vi "display_array.vi"(8 "array":i32[](array[numeric]), 11 "NXT":T1={"Hardware"="NXT", "Flattened String"=""}) -> (3 "NXT 2":T1={"Hardware"="NXT", "Flattened String"=""})   [LabVIEW 2012]
uses:
  <vilib>/NXT/Subs/LVHSConnector.ctl
  <vilib>/NXT/Dual Mode Library/Display/drawLine.vi
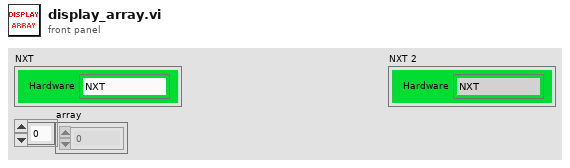
[diagram p1: front panel]
types:
  T1 = typedef "LVHSConnector.ctl" = cluster{"Hardware":string, "Flattened String":string}
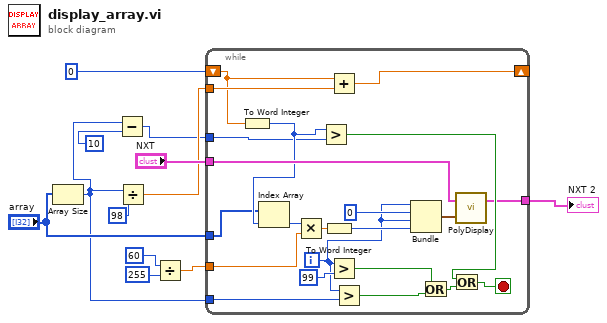
[diagram p0: block diagram]
diagram:
  n1 = Array Size(array="array") -> (size(s)=w2:i32)
  n2 = Subtract(x=w2, y=10) -> (x-y=w1:i32)
  n3 = Divide(x=w2, y=98) -> (x/y=w5:dbl)
  n4 = Divide(x=i16 60 ("Start X"), y=i16 255 ("Start X")) -> (x/y=w12:dbl)
  n5 = while {
    tunnel: [w13] -> w8
    tunnel: w12 -> [w32]
    tunnel: "NXT" -> [w29]
    tunnel: w5 -> [w28]
    shift-right: [w23] -> _
    shift-left: 0 -> [w24]
    tunnel: w2 -> [w14]
    tunnel: "array" -> [w17]
    tunnel: w1 -> [w15]
    i -> [w25]
    stop <- w19 stop-if-true
    n6 = To Word Integer(number=w24) -> (16bit integer=w22:i16)
    n7 = Index Array(array=w17, index=w22) -> (element=w16:i32)
    n8 = Multiply(x=w16, y=w32) -> (x*y=w34:dbl)
    n9 = Greater?(x=w22, y=w15) -> (0:w18:bool)
    n10 = To Word Integer(number=w34) -> (16bit integer=w31:i16)
    n11 = Add(x=w24, y=w28) -> (x+y=w23:dbl)
    n12 = Greater?(x=w25, y=99) -> (0:w21:bool)
    n13 = Greater?(x=w25, y=w14) -> (0:w26:bool)
    n14 = Bundle(w25, "Start X"=i16 0, w25, w31) -> (w30:cluster{i32, "Start X":i16, i32, i16})  [unwired: 1 in]
    n15 = Or(x=w21, y=w26) -> (x .or. y?=w20:bool)
    n16 = Or(x=w18, y=w20) -> (x .or. y?=w19:bool)
    n17 = call-poly <vilib>:"PolyDisplay.vi"("Line Parameters"=w30, "NXT"=w29) -> ("NXT"=w13:T1)  [unwired: 2 in]
  }
  "NXT 2" <- w8
